vi "Initialize with Daemon.vi"(8 "error in (no error)":errorcluster, 9 "reset device (boolean value)":bool=TRUE, 10 "Topology":string, 11 "device":refnum<k21>) -> (0 "error out":errorcluster, 3 "SLSC Switch out":refnum<class "SLSC Switch.lvclass">)   [LabVIEW 2015, in "SLSC Switch.lvlib" / "SLSC Switch.lvclass"]
doc: "Returns a session handle used to identify the switch module in all subsequent driver calls and sets the topology of the switch module."
uses:
  SLSC Switch.lvclass
  SLSC Switch.lvclass/SLSC Switch.ctl
  <vilib>/Utility/error.llb/Clear Errors.vi
  SLSC Session/Release Session.vi
  SLSC Session/SLSC Session.lvclass
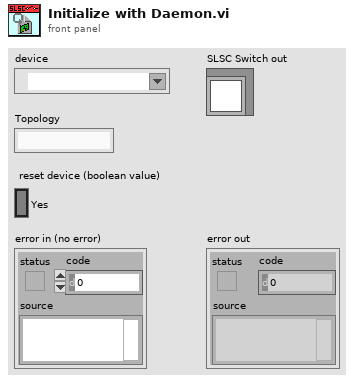
[diagram p1: front panel]
types:
  T1 = typedef "SLSC Switch.lvlib/SLSC Session.lvclass/Session Handle.ctl" = refnum<data-value>
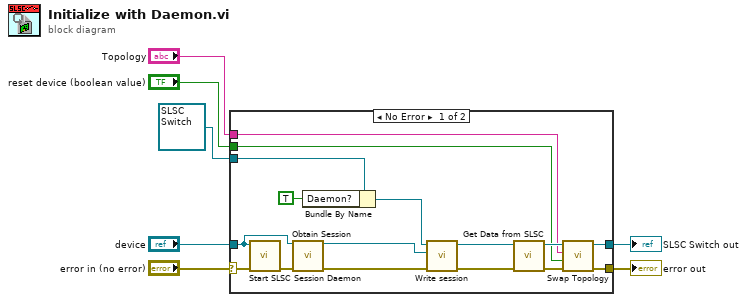
[diagram p0: block diagram]
diagram:
  n1 = case shown="No Error" "error in (no error)" {
    selector: "error in (no error)" -> [w12 w25]
    tunnel: [w17 w25] -> w6
    tunnel: refnum<class "SLSC Switch.lvclass"> refnum ("SLSC Switch in") -> [w10 w24]
    tunnel: "device" -> [w13 _]
    tunnel: "Topology" -> [w20 _]
    tunnel: "reset device (boolean value)" -> [w19 _]
    tunnel: [w16 w24] -> w1
    frame No Error {
      n2 = call "Start SLSC Session Daemon.vi"("error in (no error)"=w12, "device"=w13) -> ("error out"=w11:errorcluster)  [unwired: 9 in]
      n3 = call "Obtain Session.vi"("device"=w13, "error in (no error)"=w11) -> ("Session Handle"=w15:T1, "error out"=w14:errorcluster)  [unwired: 12 in]
      n4 = Bundle By Name(cluster=w10, "Daemon?"=TRUE) -> (w9:refnum<class "SLSC Switch.lvclass">)
      n5 = call "Write session.vi"("error in (no error)"=w14, "Session Handle"=w15, "SLSC Switch in"=w9) -> ("error out"=w23:errorcluster, "SLSC Switch out"=w22:refnum<class "SLSC Switch.lvclass">)  [unwired: 7 in]
      n6 = call "Get Data from SLSC.vi"("error in (no error)"=w23, "SLSC Switch in"=w22) -> ("error out"=w18:errorcluster, "SLSC Switch out"=w21:refnum<class "SLSC Switch.lvclass">)  [unwired: 8 in]
      n7 = call "Swap Topology.vi"("error in (no error)"=w18, "reset device (boolean value)"=w19, "Topology"=w20, "SLSC Switch in"=w21) -> ("error out"=w17:errorcluster, "SLSC Switch out"=w16:refnum<class "SLSC Switch.lvclass">)  [unwired: 6 in]
    }
    frame Error {
    }
  }
  "error out" <- w6
  "SLSC Switch out" <- w1
